vi "auto_ir_test_SL.vi"   [LabVIEW 2012, in "Mecanum Drive.lvrbt"]
uses:
  Mecanum Drive.lvrbt
  <vilib>/NXT/HiTechnic/HiTechnic Controls/HiTechnic Port.ctl
  <vilib>/NXT/Block Support/NXT_InputPort.ctl
  <vilib>/NXT/Dual Mode Library/Sound/Tone.vi
  <vilib>/NXT/Dual Mode Library/Waits/Wait_Num.vi
types:
  T1 = typedef "HiTechnic Port.ctl" = cluster{"Port":T2, "MUX Port":u8}
  T2 = typedef "NXT_InputPort.ctl" = u32
  T3 = cluster{"Direction (0-9)":i16, "Signal Strength (Array)":u8[]}
  T4 = typedef "LVHSConnector.ctl" = refnum<class "BrickReference.lvclass">
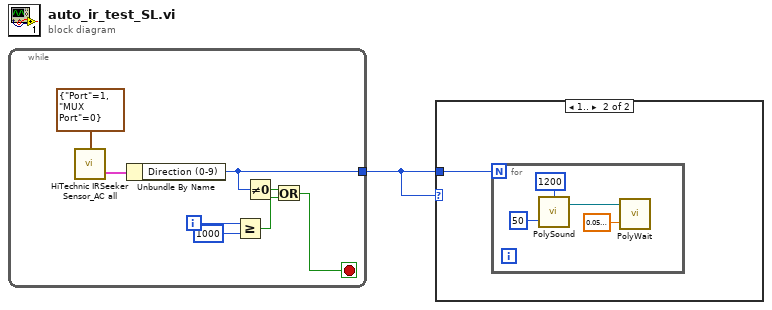
[diagram p0: block diagram]
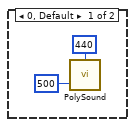
[diagram p2: hidden frame]
diagram:
  n1 = while {
    tunnel: [w7] -> w1
    i -> [w5]
    stop <- w2 stop-if-true
    n2 = call <vilib>:"HiTechnic IRSeeker Sensor_AC all.vi"("Port/MUX"=T1 {"Port"=1, "MUX Port"=0}) -> ("All Info"=w9:T3)  [unwired: 2 in, 1 out]
    n3 = Unbundle By Name(w9) -> ("Direction (0-9)"=w7:i16)
    n4 = Greater Or Equal?(x=w5, y=1000) -> (x >= y?=w3:bool)
    n5 = Not Equal To 0?(x=w7) -> (x != 0?=w6:bool)
    n6 = Or(x=w6, y=w3) -> (x .or. y?=w2:bool)
  }
  n7 = case shown="1.." w1 {
    tunnel: w1 -> [_ w12]
    frame 0, Default {
      n8 = call-poly <vilib>:"PolySound.vi"("Duration (500 ms)"=u16 500, "Tone (440 Hz)"=u16 440) -> ()  [unwired: 2 in, 1 out]
    }
    frame 1.. {
      n9 = for {
        N: w12 -> [_]
        n10 = call-poly <vilib>:"PolySound.vi"("Duration (500 ms)"=u16 50, "Tone (440 Hz)"=u16 1200) -> ("NXT/EV3"=w14:T4)  [unwired: 2 in]
        n11 = call-poly <vilib>:"PolyWait.vi"("Time (1 sec)"=sgl 0.05, "NXT/EV3"=w14) -> ()  [unwired: 2 in, 1 out]
      }
    }
  }
